vi "Console Select.vi"(7 "error in (no error)":errorcluster, 10 "Console Select":T1) -> (0 "error out":errorcluster, 2 "Console Out":string[](array[string]))   [LabVIEW 2017]
uses:
  Controls/Console Select.ctl
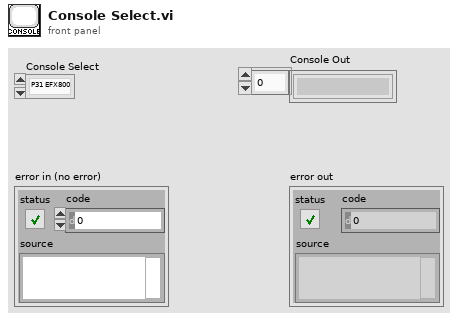
[diagram p1: front panel]
types:
  T1 = typedef "Console Select.ctl" = enum16{"P31 EFX800", "AMT", "SCL Torque"}
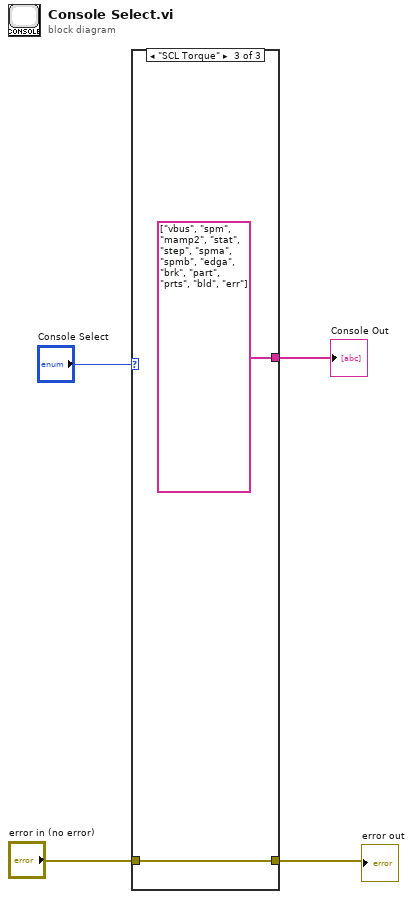
[diagram p0: block diagram]
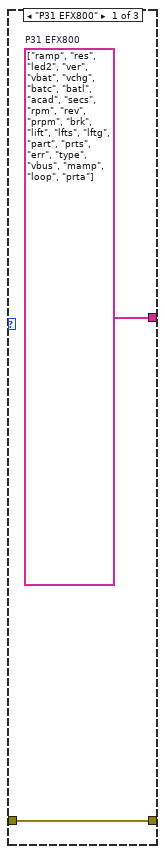
[diagram p2: hidden frame]
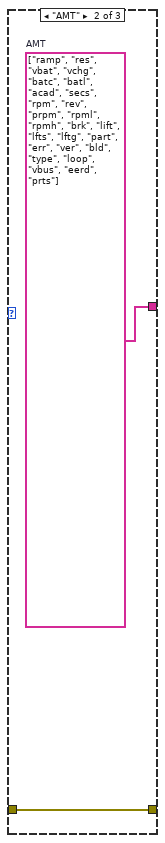
[diagram p3: hidden frame]
diagram:
  n1 = case shown="\"SCL Torque\"" "Console Select" {
    tunnel: [w6 w7 w9] -> w2
    tunnel: "error in (no error)" -> [w6 w7 w9]
    tunnel: [w5 w8 string[] ["vbus", "spm", "mamp2", "stat", "step", "spma", "spmb", "edga", "brk", "part", "prts", "bld", "err"]] -> w1
    frame "P31 EFX800" {
      w5 = string[] ["ramp", "res", "led2", "ver", "vbat", "vchg", "batc", "batl", "acad", "secs", "rpm", "rev", "prpm", "brk", "lift", "lfts", "lftg", "part", "prts", "err", "type", "vbus", "mamp", "loop", "prta"]  # P31 EFX800
    }
    frame "AMT" {
      w8 = string[] ["ramp", "res", "vbat", "vchg", "batc", "batl", "acad", "secs", "rpm", "rev", "prpm", "rpml", "rpmh", "brk", "lift", "lfts", "lftg", "part", "err", "ver", "bld", "type", "loop", "vbus", "eerd", "prts"]  # AMT
    }
    frame "SCL Torque" {
    }
  }
  "error out" <- w2
  "Console Out" <- w1
